vi "tri_cmd_lot.vi"() -> ()   [LabVIEW 2020]
uses:
  Modules/Fonction Standard/Fichier ou dossier/Cluster des Chemins.ctl
panel:
  out "Semaine":string
  out "horodatage":timestamp=timestamp(3306241065.296 s since 1904-01-01)
  in  "n° cmde":string
  out "Tableau des lots déjà emballés":string[][](array[string])
  out "Tableau historique":string[][](array[string])=[["112105740008090004", "01.01.2001 01:01:00", "55", "01234/08-01.01.01", "1", "0"], ["112105740008090006", "01.01.2001 01:01:00", "55", "56789/08-01.01.01", "3", "0"], ["112105740008090007", "01.01.2001 01:01:00", "55", "56789/08-01.01.01", "4", "0"], ["112105740008090007", "01.01.2001 01:01:00", "55", "00123/08-01.01.01", "2", "1"]]
  in  "Chemins":T1={" Admin-réseau "=path "\\\\Plz-inf-nas\\MTD_PRD_TESTS/PARAM_TESTS/PROD_Data-Admin", " XML-Réseau"=path "\\\\Plz-inf-nas\\mtd_prd_tests/PARAM_TESTS", " Résultat tests-Réseau"=path "\\\\Plz-inf-nas\\mtd_prd_tests/RESULT_TESTS", " Archive prôbleme-Réseau"=path "\\\\Plz-inf-nas\\mtd_prd_tests/RESULT_TESTS/Archives probleme reseau", " Archive Test  Local"=path "C:/Archive Test Labview"}
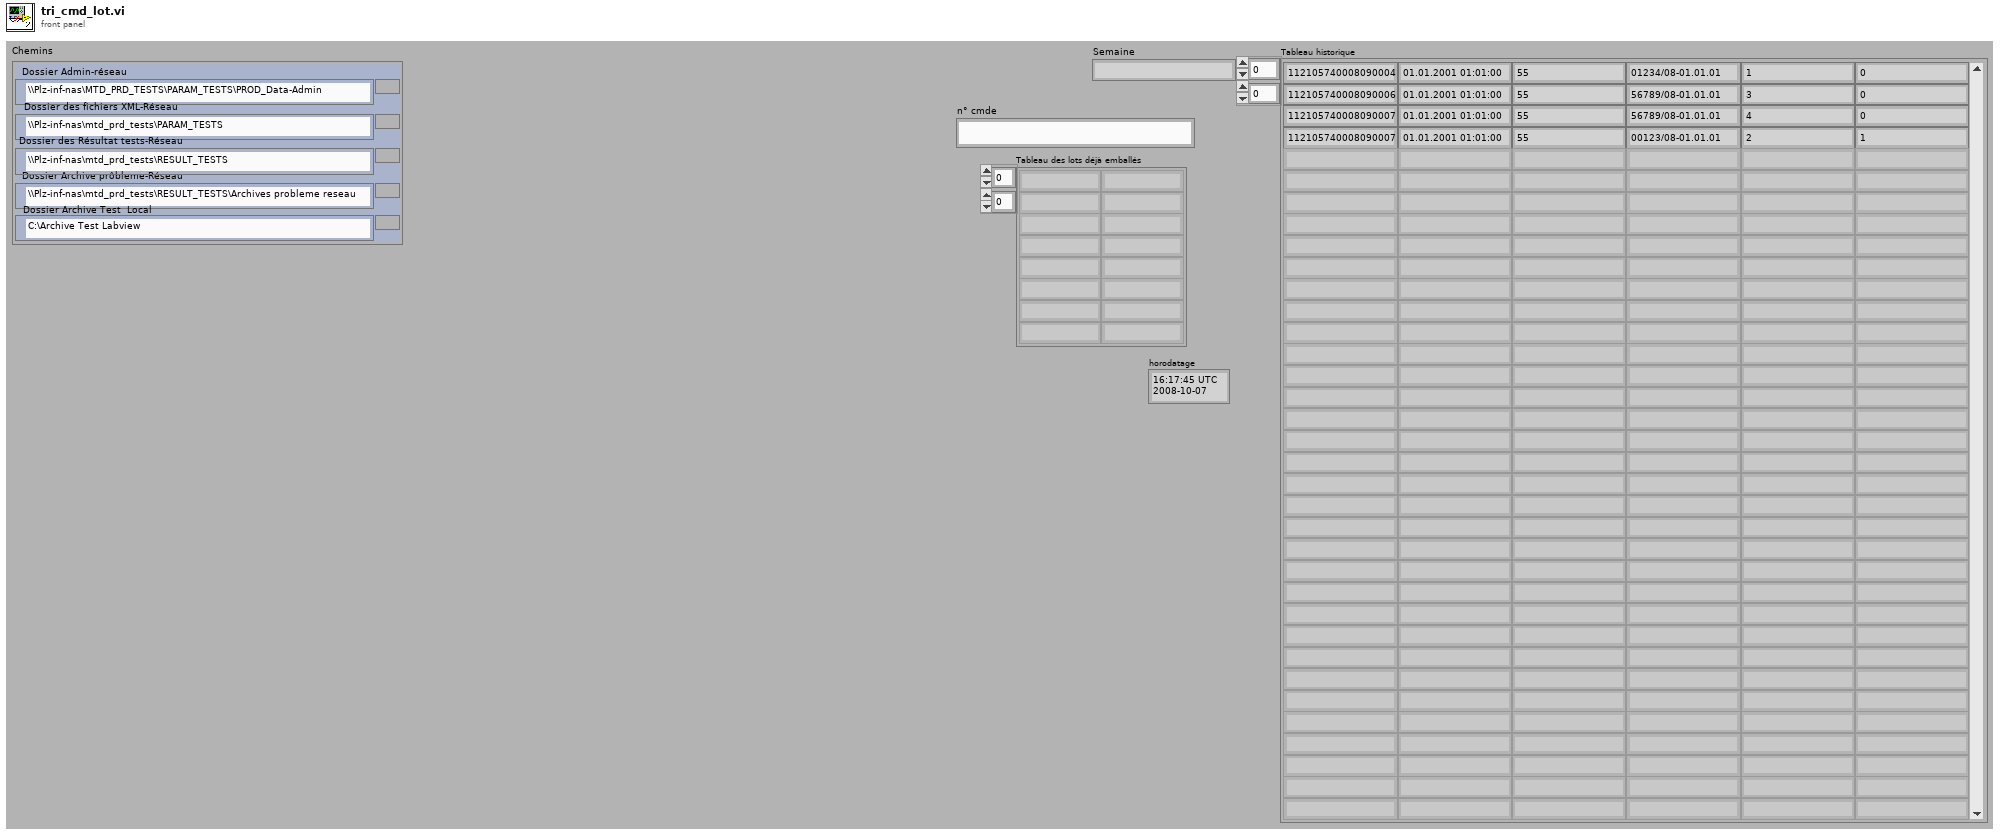
[diagram p1: front panel]
types:
  T1 = typedef "Cluster des Chemins.ctl" = cluster{" Admin-réseau ":path, " XML-Réseau":path, " Résultat tests-Réseau":path, " Archive prôbleme-Réseau":path, " Archive Test  Local":path}
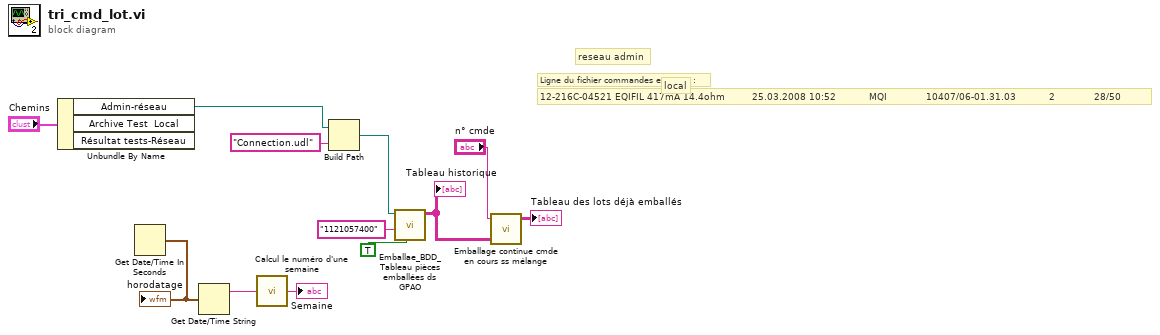
[diagram p0: block diagram]
diagram:
  # "reseau admin"
  # "local"
  # "Ligne du fichier commandes en cours :"
  # "12-216C-04521 EQIFIL 417mA 14.4ohm        \t25.03.2008 10:52          \tMQI            \t10407/06-01.31.03          \t2            \t28/50"
  n1 = Unbundle By Name("Chemins") -> ("Admin-réseau"=w11:path)  [unwired: 2 out]
  n2 = Get Date/Time In Seconds() -> (seconds since 1Jan1904=w1:timestamp)
  "horodatage" <- w1
  n3 = Get Date/Time String(seconds (now)=w1) -> (date string=w3:string)  [unwired: 2 in, 1 out]
  n4 = call "Calcul le numéro d'une semaine.vi"("chaîne de date"=w3) -> ("Semaine"=→"Semaine":string)  [unwired: 2 out]
  n5 = Build Path(base path=w11, name or relative path="Connection.udl" ("nom ou chemin relatif")) -> (appended path=w9:path)
  n6 = call "Emballae_BDD_Tableau pièces emballées ds GPAO.vi"(6:TRUE ("Activer ?"), "Code bar fixe avec indice"="1121057400", "connection information"=w9) -> ("Tableau historique"=w6:string[][])  [unwired: 6 in, 2 out]
  "Tableau historique" <- w6
  n7 = call "Emballage continue cmde en cours ss mélange.vi"(3:w6, "n° cmde"="n° cmde") -> ("Tableau des lots déjà emballés"=→"Tableau des lots déjà emballés":string[][])  [unwired: 1 in, 2 out]
